vi "Read Lump Data With REGEX.vi"(8 "Lumps Directory IN":T1[](array[typedef]), 9 "start index (0)":i32, 10 "Lump Name":string, 11 "Input U8":u8[](array[numeric])) -> (0 "Lumps Directory OUT":T1[](array[typedef]), 1 "Lump DATA OUT":u8[](array[numeric]), 2 "Found?":bool, 3 "Output U8":u8[](array[numeric]))   [LabVIEW 2017]
uses:
  Lumps.ctl
  <vilib>/regexp/Match Regular Expression.xnode
panel:
  out "x+y":i32
  out "Array":string[](array[string])
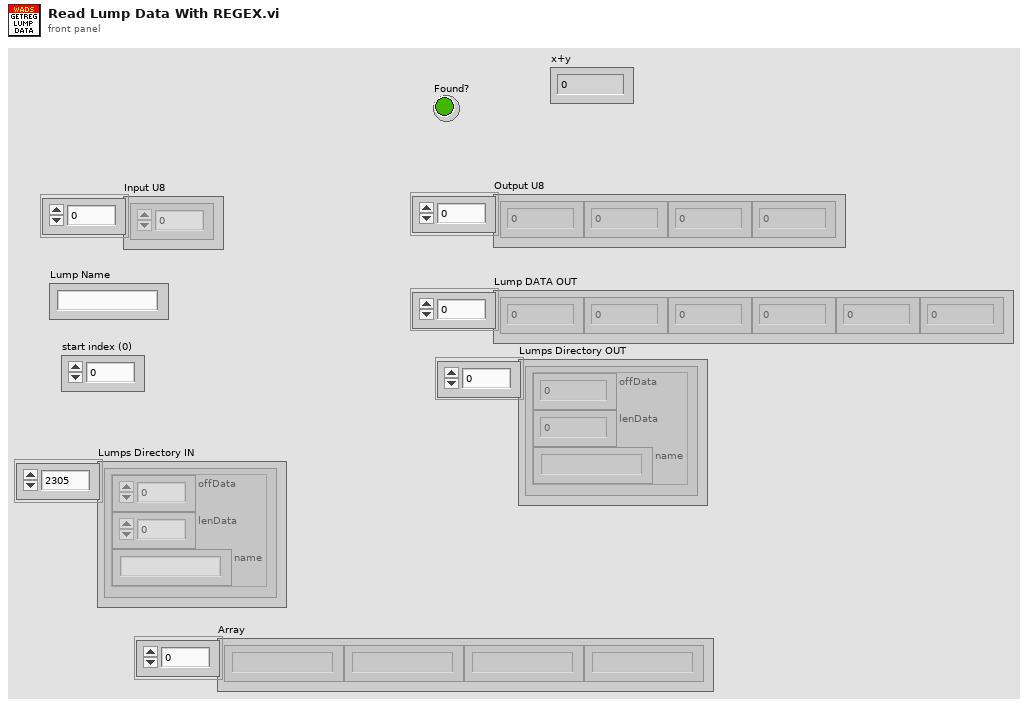
[diagram p1: front panel]
types:
  T1 = typedef "Lumps.ctl" = cluster{"offData":i32, "lenData":i32, "name":string}
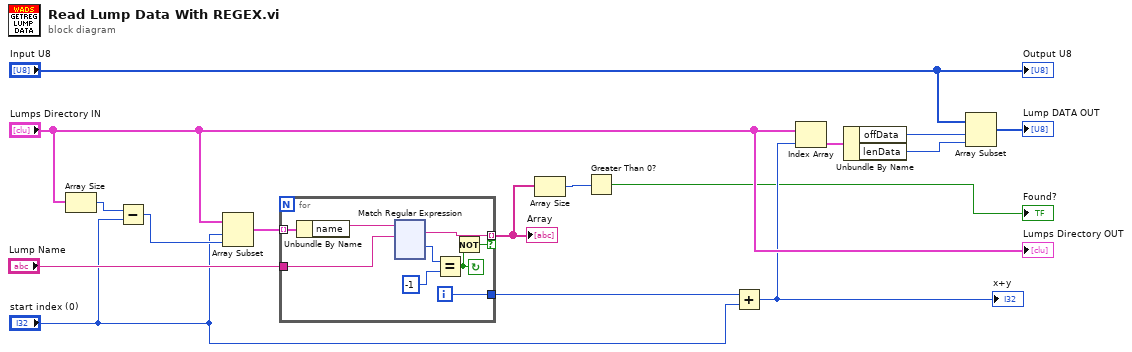
[diagram p0: block diagram]
diagram:
  n1 = Array Size(array="Lumps Directory IN") -> (size(s)=w9:i32)
  n2 = Subtract(x=w9, y="start index (0)") -> (x-y=w8:i32)
  n3 = Array Subset(array="Lumps Directory IN", index="start index (0)", length=w8) -> (w11:T1[])
  n4 = for {
    tunnel: w11 -> [w25] mode=indexing
    tunnel: [w24] -> w3 mode=indexing if=w17
    tunnel: "Lump Name" -> [w22]
    tunnel: [w21] -> w6
    i -> [w21]
    stop <- w20 continue-if-true
    n5 = Unbundle By Name(w25) -> ("name"=w19:string)
    n6 = xnode "Match Regular Expression"("input string"=w19, "regular expression"=w22) -> ("whole match"=w24:string, "offset past match"=w18:i32)  [unwired: 4 in, 3 out]
    n7 = Equal?(x=w18, y=-1) -> (x = y?=w20:bool)
    n8 = Not(x=w20) -> (.not. x?=w17:bool)
  }
  "Array" <- w3
  n9 = Array Size(array=w3) -> (size(s)=w2:i32)
  n10 = Greater Than 0?(x=w2) -> (x > 0?=→"Found?":bool)
  n11 = Add(x=w6, y="start index (0)") -> (x+y=w4:i32)
  "x+y" <- w4
  n12 = Index Array(array="Lumps Directory IN", index=w4) -> (element=w12:T1)
  n13 = Unbundle By Name(w12) -> ("offData"=w14:i32, "lenData"=w15:i32)
  n14 = Array Subset(array="Input U8", index=w14, length=w15) -> (→"Lump DATA OUT":u8[])
  "Output U8" <- "Input U8"
  "Lumps Directory OUT" <- "Lumps Directory IN"
